vi "AlliGator Logistic Square Gated IRF Fit Result File String.vi"(8 "error in (no error)":errorcluster, 9 "Delta Best Fit Parameters":dbl[](array[numeric]), 10 "Fit Output":T1={"best nonlinear fit"=[], "best fit parameters"=[], "R^2"=0.0, "RMSE"=0.0, "error out"={"status"=FALSE, "code"=0, "source"=""}, "Fitting Method"=enum."Least Square", "number of function calls"=0, "number of iterations"=0, "covariance"=[], "Chi 2"=0.0, "DOF"=0, "Fit Convergence Criterion"=enum."Continue", "Fitting Algorithm"=enum."Levenberg-Marquardt", "Weighted Fit"=FALSE, "Gradient"=0.0, "|Delta Chi 2|"=0.0, "|Delta Chi 2|/Chi 2"=0.0, "Max |Delta a| /|a|"=0.0, "Lambda"=-1.0, "RSS"=0.0, "AIC"=0.0, "BIC"=0.0, "Max number of function calls"=0, "Max number of iterations"=0, "IRF"={"X Array"=[], "Y Array"=[]}, "IRF Normalization Factor"=0.0, "Decay Normalization Factor"=0.0}, 11 "ROI Descriptor":T7 {"Contours"."Type" items=["No Selection", "Point", "Line", "Rectangle", "Oval", "Polygon", "Freehand Region", "Annulus", "Unused2", "Unused3", "Broken Line", "Freehand Line", "Rotated Rectangle"]}) -> (0 "error out":errorcluster, 3 "Result String":string, 5 "Header String":string="ROI_x\tROI_y\tAL\tAL_err\tAU\tAU_err\tx0R\tx0R_err\tdxR\tdxR_err\tx0F\tx0F_err\tdxF\tdxF_err\tR^2\tRMSE\tMethod\tCalls\tIterations")   [LabVIEW 2021, in "AlliGator Scripts.lvlib"]
doc: "Builds string containing the output of a logistic square gate fit."
uses:
  AlliGator Scripts.lvlib
  Fits/Non-linear Fit Output v3.ctl
  Fits/Nonlinear Fit Method.ctl
  <vilib>/Analysis/Matrix/Datatypes/RealMatrix.ctl
  Fits/Convergence Criteria.ctl
  Fits/Non-linear Fitting Algorithm.ctl
  Graphs/XY Graph/XY Plot Data.ctl
  <vilib>/Analysis/Matrix/NI_Matrix.lvlib
  Fits/Fits.lvlib
  Graphs/XY Graph/XY Graph Add-Ons.lvlib
panel:
  # "see the AlliGator License on the block diagram (Ctrl+E or Window:Show Block Diagram)"
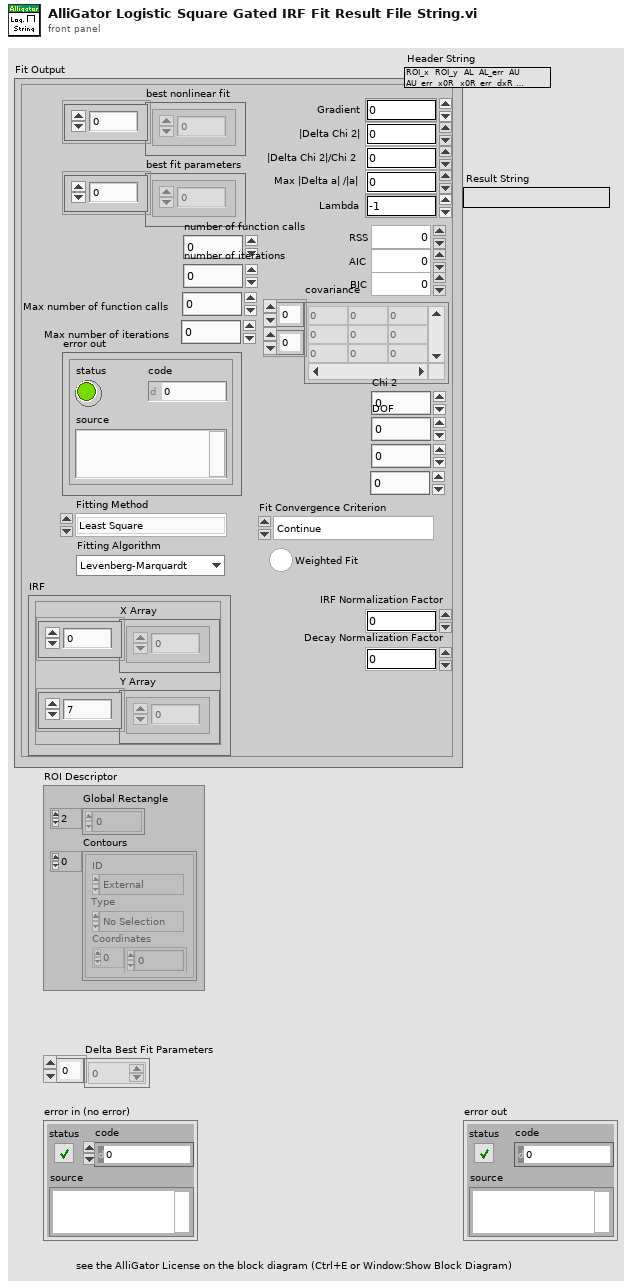
[diagram p1: front panel]
types:
  T1 = typedef "Fits.lvlib/Non-linear Fit Output v3.ctl" = cluster{"best nonlinear fit":dbl[], "best fit parameters":dbl[], "R^2":dbl, "RMSE":dbl, "error out":errorcluster, "Fitting Method":T2, "number of function calls":i32, "number of iterations":i32, "covariance":T3, "Chi 2":dbl, "DOF":i32, "Fit Convergence Criterion":T4, "Fitting Algorithm":T5, "Weighted Fit":bool, "Gradient":dbl, "|Delta Chi 2|":dbl, "|Delta Chi 2|/Chi 2":dbl, "Max |Delta a| /|a|":dbl, "Lambda":dbl, "RSS":dbl, "AIC":dbl, "BIC":dbl, "Max number of function calls":i32, "Max number of iterations":i32, "IRF":T6, "IRF Normalization Factor":dbl, "Decay Normalization Factor":dbl}
  T2 = typedef "Fits.lvlib/Nonlinear Fit Method.ctl" = enum16{"Least Square", "Least Absolute Residual", "Bisquare", "MLE"}
  T3 = typedef "NI_Matrix.lvlib/RealMatrix.ctl" = dbl[][]
  T4 = typedef "Fits.lvlib/Convergence Criteria.ctl" = enum16{"Continue", "Tolerances Exceeded", "Max Time Exceeded", "Max Iterations Exceeded", "Max Function Evaluations Exceeded", "Scale Range Exceeded"}
  T5 = typedef "Fits.lvlib/Non-linear Fitting Algorithm.ctl" = enum16{"Levenberg-Marquardt", "Trust-Region Dogleg"}
  T6 = typedef "XY Graph Add-Ons.lvlib/XY Plot Data.ctl" = cluster{"X Array":dbl[], "Y Array":dbl[]}
  T7 = typedef "ROI Descriptor" = cluster{"Global Rectangle":i32[], "Contours":cluster{"ID":enum32{"External", "Internal"}, "Type":u32, "Coordinates":i32[]}[]}
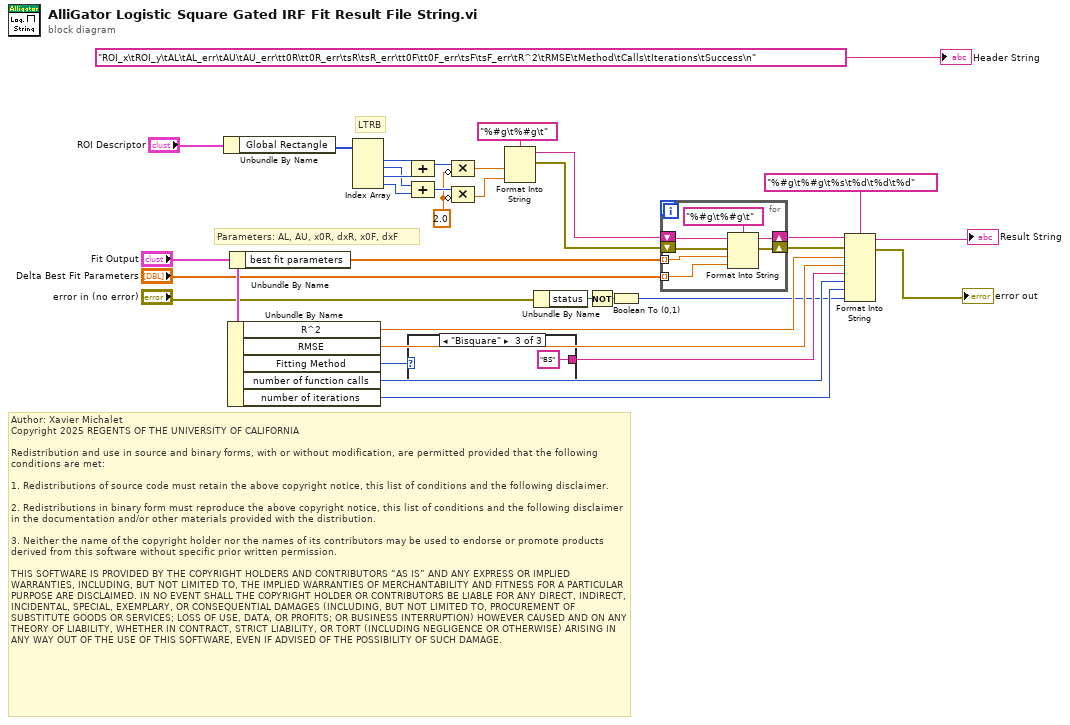
[diagram p0: block diagram]
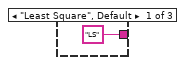
[diagram p2: hidden frame]
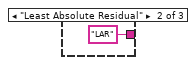
[diagram p3: hidden frame]
diagram:
  w11 = 2.0 ("value")
  # "Author: Xavier Michalet\nCopyright 2025 REGENTS OF THE UNIVERSITY OF CALIFORNIA\n\nRedistribution and use in source and binary forms, with or without modification, are permitted provided that the following conditions are met:\n\n1. Redistributions of source code must retain the above copyright notice, this list of conditions and the following disclaimer.\n\n2. Redistributions in binary form must reproduce the above copyright notice, this list of conditions and the following disclaimer in the documentation and/or other materials provided with the distribution.\n\n3. Neither the name of the copyright holder nor the names of its contributors may be used to endorse or promote products derived from this software without specific prior written permission.\n\nTHIS SOFTWARE IS PROVIDED BY THE COPYRIGHT HOLDERS AND CONTRIBUTORS “AS IS” AND ANY EXPRESS OR IMPLIED WARRANTIES, INCLUDING, BUT NOT LIMITED TO, THE IMPLIED WARRANTIES OF MERCHANTABILITY AND FITNESS FOR A PARTICULAR PURPOSE ARE DISCLAIMED. IN NO EVENT SHALL THE COPYRIGHT HOLDER OR CONTRIBUTORS BE LIABLE FOR ANY DIRECT, INDIRECT, INCIDENTAL, SPECIAL, EXEMPLARY, OR CONSEQUENTIAL DAMAGES (INCLUDING, BUT NOT LIMITED TO, PROCUREMENT OF SUBSTITUTE GOODS OR SERVICES; LOSS OF USE, DATA, OR PROFITS; OR BUSINESS INTERRUPTION) HOWEVER CAUSED AND ON ANY THEORY OF LIABILITY, WHETHER IN CONTRACT, STRICT LIABILITY, OR TORT (INCLUDING NEGLIGENCE OR OTHERWISE) ARISING IN ANY WAY OUT OF THE USE OF THIS SOFTWARE, EVEN IF ADVISED OF THE POSSIBILITY OF SUCH DAMAGE."
  # "LTRB"
  # "Parameters: AL, AU, x0R, dxR, x0F, dxF"
  n1 = Unbundle By Name("ROI Descriptor") -> ("Global Rectangle"=w28:i32[])
  n2 = Unbundle By Name("Fit Output") -> ("R^2"=w6:dbl, "RMSE"=w5:dbl, "Fitting Method"=w17:T2, "number of function calls"=w15:i32, "number of iterations"=w14:i32)
  n3 = Unbundle By Name("Fit Output") -> ("best fit parameters"=w8:dbl[])
  n4 = Index Array(array=w28) -> (element #1=w27:i32, element #2=w24:i32, element #3=w26:i32, element #4=w25:i32)  [unwired: 4 in]
  n5 = case shown="\"Bisquare\"" w17 {
    tunnel: ["LS" ("input 3") "LAR" ("input 3") "BS" ("input 3")] -> w16
    frame "Least Square", Default {
    }
    frame "Least Absolute Residual" {
    }
    frame "Bisquare" {
    }
  }
  n6 = Compound Arithmetic op=ADD(w27, w26) -> (w13:i32)
  n7 = Compound Arithmetic op=ADD(w24, w25) -> (w12:i32)
  n8 = Compound Arithmetic op=MULTIPLY(w13, invert w11) -> (w10:dbl)
  n9 = Compound Arithmetic op=MULTIPLY(w12, invert w11) -> (w9:dbl)
  n10 = Format Into String(format string="%#g\t%#g\t", w10, w9) -> (resulting string=w21:string, error out=w22:errorcluster)  [unwired: 2 in]
  n11 = Unbundle By Name("error in (no error)") -> ("status"=w3:bool)
  n12 = Not(x=w3) -> (.not. x?=w2:bool)
  n13 = Boolean To (0,1)(Boolean=w2) -> (0, 1=w1:i16)
  n14 = for {
    tunnel: w8 -> [w42] mode=indexing
    tunnel: "Delta Best Fit Parameters" -> [w41] mode=indexing
    shift-right: [w39] -> w20
    shift-left: w21 -> [w40]
    shift-right: [w38] -> w19
    shift-left: w22 -> [w37]
    n15 = Format Into String(format string="%#g\t%#g\t", initial string=w40, error in=w37, w42, w41) -> (resulting string=w39:string, error out=w38:errorcluster)
  }
  n16 = Format Into String(format string="%#g\t%#g\t%s\t%d\t%d\t%d", initial string=w20, error in=w19, w6, w5, w16, w15, w14, w1) -> (resulting string=→"Result String":string, error out=→"error out":errorcluster)
  "Header String" <- "ROI_x\tROI_y\tAL\tAL_err\tAU\tAU_err\tt0R\tt0R_err\tsR\tsR_err\tt0F\tt0F_err\tsF\tsF_err\tR^2\tRMSE\tMethod\tCalls\tIterations\tSuccess\n" ("format string")
